vi "sv_Insert Swept RMS Values.vi"(8 "scaled measurements in":T1 {"harmonic components [ratio]" format="%.2f"; "THD [ratio]" format="%.2f"; "FRF Measurements"."Im [response]" format="%.2f"; "FRF Measurements"."Re [response]" format="%.2f"; "FRF Measurements"."Im [stimulus]" format="%.2f"; "FRF Measurements"."Re [stimulus]" format="%.2f"; "RMS response" format="%.2f"; "RMS stimulus" format="%.2f"}, 10 "AI freq index":i32, 11 "measurements in":T2 {"scaled response magnitude" format="%.3f"; "Harm[]" format="%.2f"; "THD" format="%.2f"; "Im [response]" format="%.2f"; "Re [response]" format="%.2f"; "Im [stimulus]" format="%.2f"; "Re [stimulus]" format="%.2f"; "RMS response" format="%.2f"; "RMS stimulus" format="%.2f"}) -> (0 "scaled measurements in":T1 {"harmonic components [ratio]" format="%.2f"; "THD [ratio]" format="%.2f"; "FRF Measurements"."Im [response]" format="%.2f"; "FRF Measurements"."Re [response]" format="%.2f"; "FRF Measurements"."Im [stimulus]" format="%.2f"; "FRF Measurements"."Re [stimulus]" format="%.2f"; "RMS response" format="%.2f"; "RMS stimulus" format="%.2f"}, 2 "dup AI freq index":i32, 3 "measurements out":T2 {"scaled response magnitude" format="%.3f"; "Harm[]" format="%.2f"; "THD" format="%.2f"; "Im [response]" format="%.2f"; "Re [response]" format="%.2f"; "Im [stimulus]" format="%.2f"; "Re [stimulus]" format="%.2f"; "RMS response" format="%.2f"; "RMS stimulus" format="%.2f"})   [LabVIEW 2017, in "SoundVib_SweptSine.lvlib"]
uses:
  <vilib>/addons/Sound and Vibration/svt_Swept Sine/SoundVib_SweptSine.lvlib
  <vilib>/addons/Sound and Vibration/svt_Swept Sine/subVIs/sv_Swept Sine Measurements.ctl
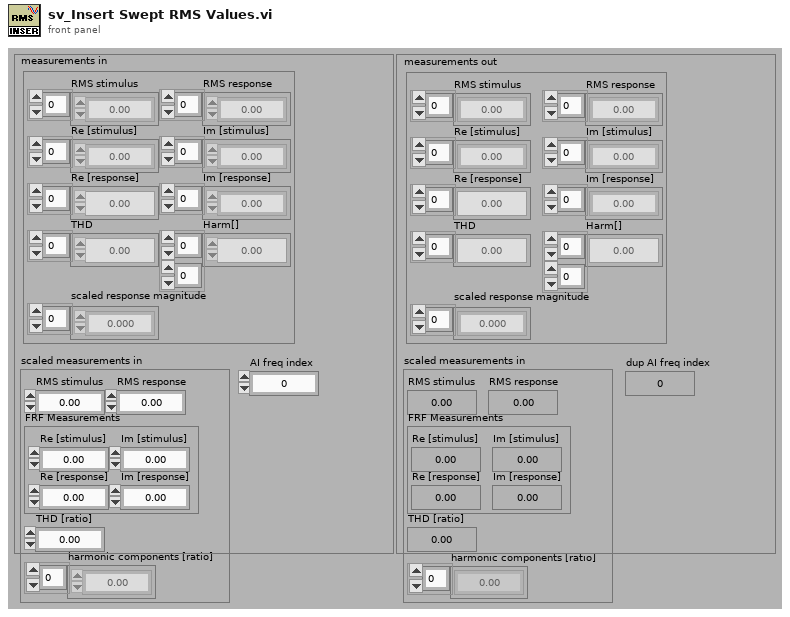
[diagram p1: front panel]
types:
  T1 = cluster{"RMS stimulus":dbl, "RMS response":dbl, "FRF Measurements":cluster{"Re [stimulus]":dbl, "Im [stimulus]":dbl, "Re [response]":dbl, "Im [response]":dbl}, "THD [ratio]":dbl, "harmonic components [ratio]":dbl[]}
  T2 = typedef "SoundVib_SweptSine.lvlib/sv_Swept Sine Measurements.ctl" = cluster{"RMS stimulus":dbl[], "RMS response":dbl[], "Re [stimulus]":dbl[], "Im [stimulus]":dbl[], "Re [response]":dbl[], "Im [response]":dbl[], "THD":dbl[], "Harm[]":dbl[][], "scaled response magnitude":dbl[]}
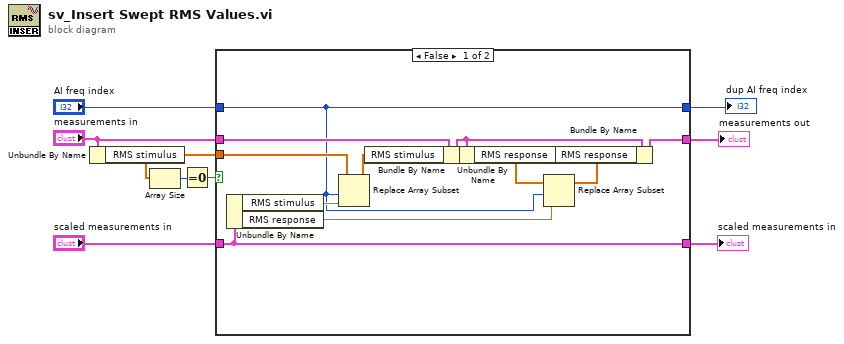
[diagram p0: block diagram]
diagram:
  n1 = Unbundle By Name("measurements in") -> ("RMS stimulus"=w2:dbl[])
  n2 = Array Size(array=w2) -> (size(s)=w4:i32)
  n3 = Equal To 0?(x=w4) -> (x = 0?=w3:bool)
  n4 = case shown="False" w3 {
    tunnel: "measurements in" -> [w16 w23]
    tunnel: [w14 w23] -> w8
    tunnel: w2 -> [w15 _]
    tunnel: "scaled measurements in" -> [w11 w22]
    tunnel: [w11 w22] -> w6
    tunnel: "AI freq index" -> [w10 w21]
    tunnel: [w10 w21] -> w1
    frame False {
      n5 = Unbundle By Name(w11) -> ("RMS stimulus"=w12:dbl, "RMS response"=w13:dbl)
      n6 = Replace Array Subset(array=w15, new element=w12, index=w10) -> (w17:dbl[])
      n7 = Bundle By Name(cluster=w16, "RMS stimulus"=w17) -> (w19:T2)
      n8 = Unbundle By Name(w19) -> ("RMS response"=w18:dbl[])
      n9 = Replace Array Subset(array=w18, new element=w13, index=w10) -> (w20:dbl[])
      n10 = Bundle By Name(cluster=w19, "RMS response"=w20) -> (w14:T2)
    }
    frame True {
    }
  }
  "measurements out" <- w8
  "scaled measurements in" <- w6
  "dup AI freq index" <- w1
